vi "ConditionalString.vi"(1 "String in":string) -> (0 "Stop?":bool)   [LabVIEW 2017]
doc: "Displays the value of the string and allows conditional breakpoints."
panel:
  in  "Tab Control":enum32{"Data", "Condition"}(tab)
  out "String out":string
  in  "Conditional String":string
  in  "Pause If:":u16(ring) items=["<None>", "Ends with", "Equals", "Not Equal", "Starts with", "Contains", "Matches pattern"]
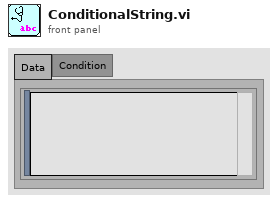
[diagram p1: front panel]
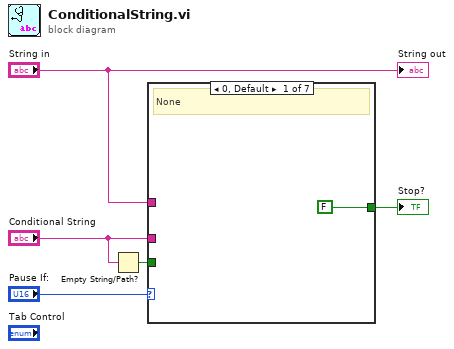
[diagram p0: block diagram]
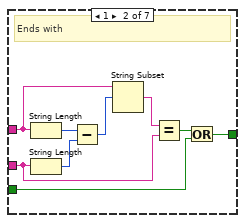
[diagram p2: hidden frame]
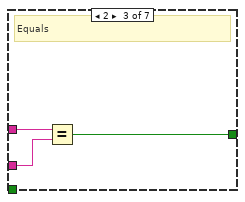
[diagram p3: hidden frame]
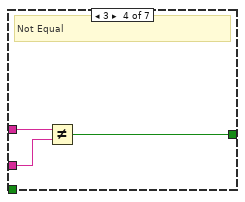
[diagram p4: hidden frame]
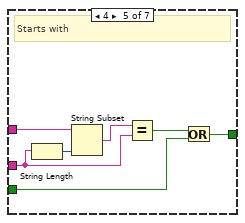
[diagram p5: hidden frame]
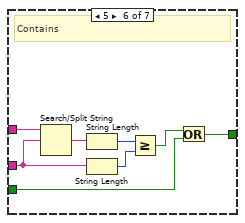
[diagram p6: hidden frame]
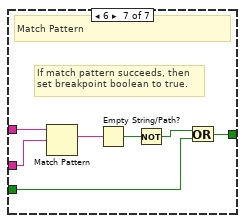
[diagram p7: hidden frame]
diagram:
  n1 = Empty String/Path?(string/path="Conditional String") -> (empty?=w3:bool)
  n2 = case shown="0, Default" "Pause If:" {
    tunnel: "String in" -> [_ w11 w18 w21 w25 w36 w43]
    tunnel: "Conditional String" -> [_ w9 w17 w20 w22 w35 w42]
    tunnel: [FALSE w14 w16 w19 w27 w29 w37] -> w2
    tunnel: w3 -> [_ w8 _ _ w23 w30 w39]
    frame 0, Default {
      # "None"
    }
    frame 1 {
      # "Ends with"
      n3 = String Length(string=w11) -> (length=w13:i32)
      n4 = String Length(string=w9) -> (length=w12:i32)
      n5 = Subtract(x=w13, y=w12) -> (x-y=w7:i32)
      n6 = String Subset(string=w11, offset (0)=w7) -> (substring=w10:string)  [unwired: 1 in]
      n7 = Equal?(x=w10, y=w9) -> (x = y?=w15:bool)
      n8 = Or(x=w15, y=w8) -> (x .or. y?=w14:bool)
    }
    frame 2 {
      # "Equals"
      n9 = Equal?(x=w18, y=w17) -> (x = y?=w16:bool)
    }
    frame 3 {
      # "Not Equal"
      n10 = Not Equal?(x=w21, y=w20) -> (x != y?=w19:bool)
    }
    frame 4 {
      # "Starts with"
      n11 = String Length(string=w22) -> (length=w26:i32)
      n12 = String Subset(string=w25, length (rest)=w26) -> (substring=w24:string)  [unwired: 1 in]
      n13 = Equal?(x=w24, y=w22) -> (x = y?=w28:bool)
      n14 = Or(x=w28, y=w23) -> (x .or. y?=w27:bool)
    }
    frame 5 {
      # "Contains"
      n15 = Search/Split String(string=w36, search string/char (-)=w35) -> (match + rest of string=w34:string)  [unwired: 1 in, 2 out]
      n16 = String Length(string=w34) -> (length=w33:i32)
      n17 = String Length(string=w35) -> (length=w32:i32)
      n18 = Greater Or Equal?(x=w33, y=w32) -> (x >= y?=w31:bool)
      n19 = Or(x=w31, y=w30) -> (x .or. y?=w29:bool)
    }
    frame 6 {
      # "If match pattern succeeds, then\nset breakpoint boolean to true."
      # "Match Pattern"
      n20 = Match Pattern(string=w43, regular expression=w42) -> (match substring=w41:string)  [unwired: 1 in, 3 out]
      n21 = Empty String/Path?(string/path=w41) -> (empty?=w40:bool)
      n22 = Not(x=w40) -> (.not. x?=w38:bool)
      n23 = Or(x=w38, y=w39) -> (x .or. y?=w37:bool)
    }
  }
  "Stop?" <- w2
  "String out" <- "String in"
